vi "phase_tracking_HOST.vi"() -> ()   [LabVIEW 2017]
uses:
  <vilib>/userdefined/High Color/nirio_resource_hc.ctl
  <vilib>/rvi/Analysis/host/Butterworth/config/Butterworth Filter Order.ctl
  <vilib>/rvi/Analysis/host/Butterworth/config/Butterworth Filter Type.ctl
  <vilib>/FPGAPlugInAG/PCIe-7841R/niLvFpga_Open_PCIe-7841R.vi
  <vilib>/rvi/interface/common/dynamic/niFpgaDynamicAddResources.vi
  <vilib>/FPGAPlugInAG/Dynamic/niLvFpga_Run_Dynamic.vi
  <vilib>/rvi/Analysis/host/Butterworth/config/BwScaledCoefficients.vi
  <vilib>/Utility/error.llb/Error Cluster From Error Code.vi
  <vilib>/rvi/errors/niLvFpgaAdjustHostInterfaceError.vi
  <vilib>/FPGAPlugInAG/Dynamic/niLvFpga_Close_Dynamic.vi
  <vilib>/rvi/interface/nirviOpenFPGA/nirviOpenFPGA.xnode
  FPGA Bitfiles/phasetracking_FPGATarget_phasetracking_sogMn92qpVI.lvbitx
  <vilib>/rvi/interface/nirviMethod/nirviMethod.xnode
  <vilib>/rvi/Analysis/host/Butterworth/XNode/ButterworthCoefficients.xnode
  <vilib>/rvi/interface/nirviReadWriteControl/nirviReadWriteControl.xnode
  <vilib>/rvi/interface/nirviCloseFPGA/nirviCloseFPGA.xnode
  <vilib>/rvi/interface/Simulation/niFpgaSimulationCallBeginRW.vi
  NiFpgaLv.dll
  <vilib>/rvi/Analysis/host/Public/NI_FpgaMspHost.lvlib
panel:
  out "Phi Full (FPGA)":dbl(graph)
  out "Phi Full (Host)":dbl(graph)
  out "Phi":dbl(graph)
  in  "Update Freq":dbl format="%#_13g"
  in  "Delay (samples)":u16
  in  "RIO Device":T1
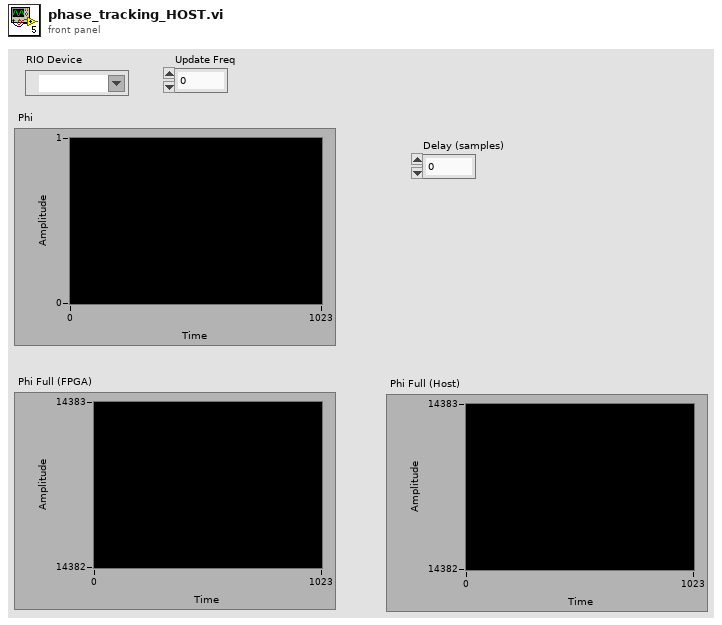
[diagram p1: front panel]
types:
  T1 = typedef "nirio_resource_hc.ctl" = tag
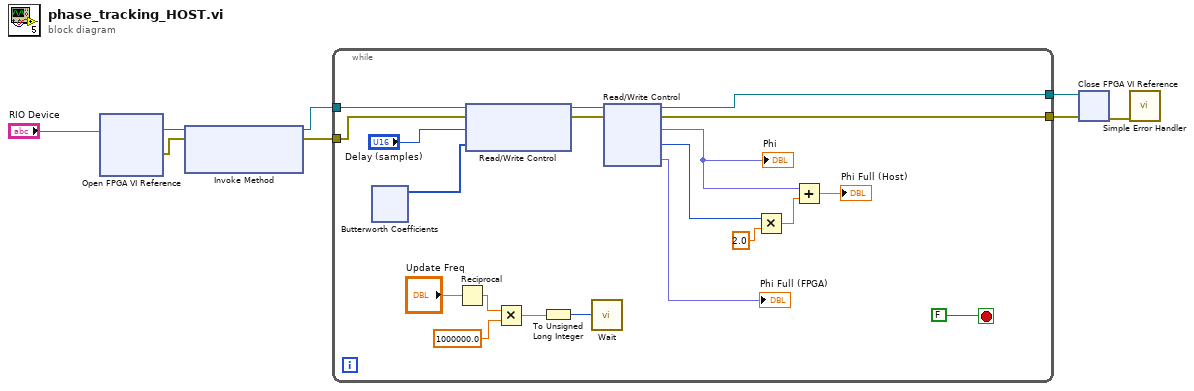
[diagram p0: block diagram]
diagram:
  n1 = xnode "Open FPGA VI Reference"("resource name"="RIO Device") -> ("FPGA VI Reference Out"=w8:refnum<k20>, "error out"=w7:errorcluster)  [unwired: 1 in]
  n2 = xnode "Invoke Method"("FPGA VI Reference In"=w8, "error in"=w7) -> ("FPGA VI Reference Out"=w6:refnum<k20>, "error out"=w5:errorcluster)  [unwired: 1 in]
  n3 = while {
    tunnel: [w27] -> w4
    tunnel: w6 -> [w25]
    tunnel: w5 -> [w23]
    tunnel: [w26] -> w3
    stop <- FALSE stop-if-true
    n4 = xnode "Butterworth Coefficients"() -> ("scaled coefficients"=w9:i32[])  [unwired: 3 in, 1 out]
    n5 = Reciprocal(x="Update Freq") -> (1/x=w19:dbl)
    n6 = xnode "Read/Write Control"("FPGA VI Reference In"=w25, "error in"=w23, "delay"="Delay (samples)", "phase_filt_coeffs"=w9) -> ("FPGA VI Reference Out"=w24:refnum<k20>, "error out"=w22:errorcluster)
    n7 = Multiply(x=w19, y=1000000.0) -> (x*y=w17:dbl)
    n8 = To Unsigned Long Integer(number=w17) -> (unsigned 32bit integer=w16:u32)
    n9 = call "Wait"("Count(uSec)"=w16) -> ()  [unwired: 1 out]
    n10 = xnode "Read/Write Control"("FPGA VI Reference In"=w24, "error in"=w22) -> ("FPGA VI Reference Out"=w26:refnum<k20>, "error out"=w27:errorcluster, "Phi"=w15:fxp<+/-,16,2>, "n"=w11:i16, "Phi Full"=→"Phi Full (FPGA)":fxp<+/-,32,18>)
    "Phi" <- w15
    n11 = Multiply(x=w11, y=2.0) -> (x*y=w12:dbl)
    n12 = Add(x=w15, y=w12) -> (x+y=→"Phi Full (Host)":dbl)
  }
  n13 = xnode "Close FPGA VI Reference"("FPGA VI Reference In"=w3, "error in"=w4) -> ("error out"=w2:errorcluster)
  n14 = call <vilib>:"Simple Error Handler.vi"("error in (no error)"=w2) -> ()  [unwired: 4 in, 5 out]
